vi "Example - Simple Test.vi"   [LabVIEW 2017]
uses:
  UUT_class/UUT.lvclass
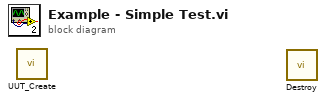
[diagram p0: block diagram]
diagram:
  n1 = call "UUT_Create.vi"() -> ()  [unwired: 18 in, 2 out]
  n2 = call-dynamic "Destroy.vi"() -> ()  [unwired: 18 in, 2 out]
